vi "Read FPGA Setting.vi"(8 "error in (no error)":errorcluster, 11 "FPGA configuration in":refnum<class "FPGA configuration.lvclass">) -> (0 "error out":errorcluster, 2 "FPGA Setting":T1={"Numeric"=0.5, "Combo"="", "String"="", "Boolean"=FALSE} {"Numeric" format="%#_f"}, 3 "FPGA configuration out":refnum<class "FPGA configuration.lvclass">)   [LabVIEW 2025, in "FPGA.lvlib" / "FPGA configuration.lvclass"]
uses:
  FPGA configuration.lvclass
  FPGA Setting.ctl
  FPGA configuration.lvclass/FPGA configuration.ctl
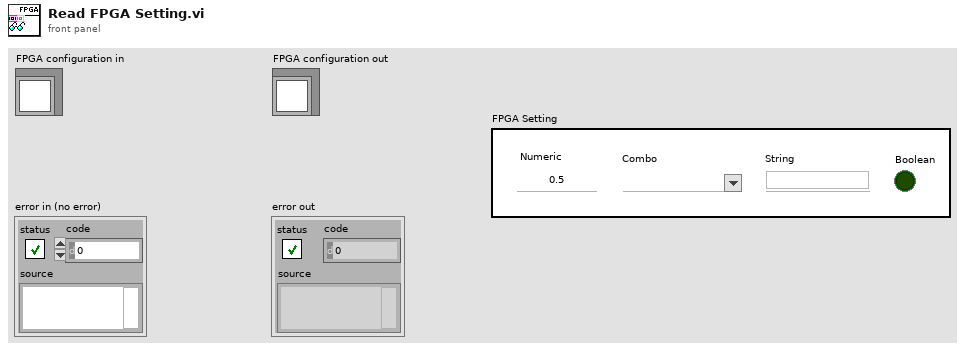
[diagram p1: front panel]
types:
  T1 = typedef "FPGA.lvlib/FPGA configuration.lvclass/FPGA Setting.ctl" = cluster{"Numeric":dbl, "Combo":string, "String":string, "Boolean":bool}
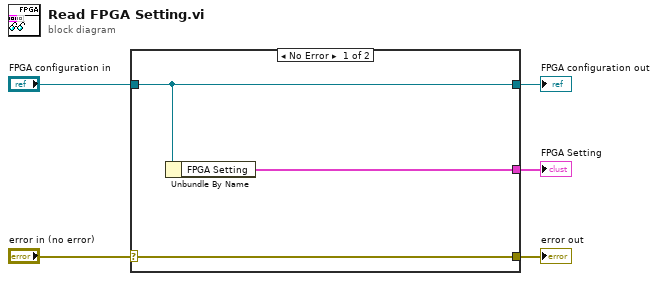
[diagram p0: block diagram]
diagram:
  n1 = case shown="No Error" "error in (no error)" {
    selector: "error in (no error)" -> [w8 w9]
    tunnel: [w8 w9] -> w4
    tunnel: [w7 w10] -> w2
    tunnel: "FPGA configuration in" -> [w7 w10]
    tunnel: [w6 _] -> w1
    frame No Error {
      n2 = Unbundle By Name(w7) -> ("FPGA Setting"=w6:T1)
    }
    frame Error {
    }
  }
  "error out" <- w4
  "FPGA configuration out" <- w2
  "FPGA Setting" <- w1
